vi "数组分解(二维转16行).vi"(1 "输入数组":string[][](array[string])) -> (0 "输出数组":string[][](array[string]))   [LabVIEW 2013]
panel:
  out "子数组":string[][](array[string])
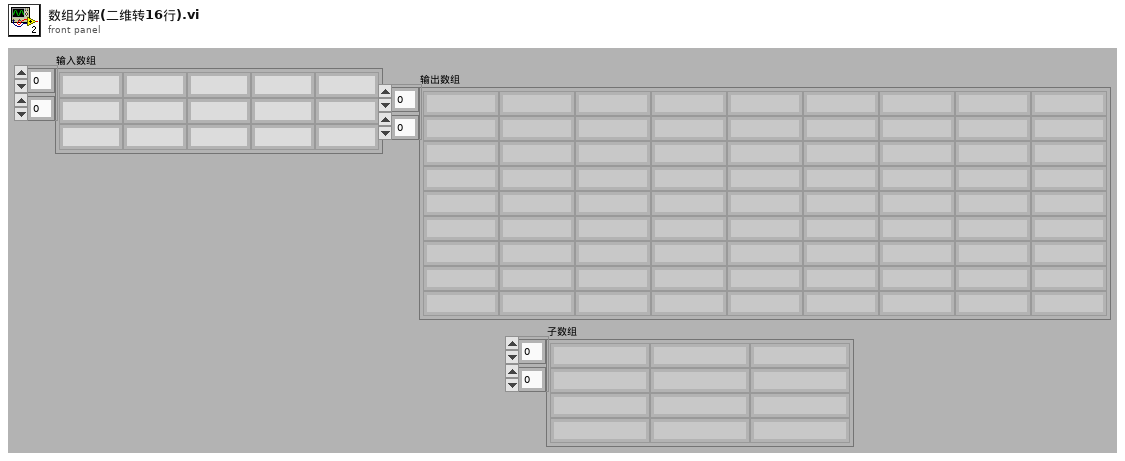
[diagram p1: front panel]
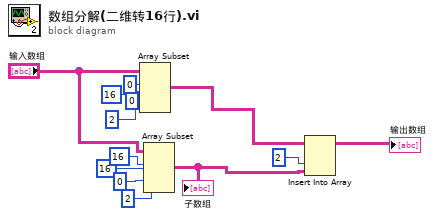
[diagram p0: block diagram]
diagram:
  n1 = Array Subset(array="输入数组", index (row)=0 ("索引"), length (row)=16 ("长度"), index (col)=0 ("索引"), length (col)=2 ("长度")) -> (w8:string[][])
  n2 = Array Subset(array="输入数组", index (row)=16 ("索引"), length (row)=16 ("长度"), index (col)=0 ("索引"), length (col)=2 ("长度")) -> (w11:string[][])
  "子数组" <- w11
  n3 = Insert Into Array(array=w8, index (col)=2 ("禁用的索引 (列)"), new element=w11) -> (→"输出数组":string[][])  [unwired: 1 in]
